vi "Shutdown.vi"(8 "error in (no error)":errorcluster, 11 "Nominal Streaming in":refnum<class "Stream.lvclass">) -> (0 "error out":errorcluster, 3 "Nominal Streaming out":refnum<class "Stream.lvclass">)   [LabVIEW 2020, in "Nominal Streaming.lvlib" / "Stream.lvclass"]
uses:
  Stream.lvclass
  Stream.lvclass/Stream.ctl
  bin/lib_nominal-streaming-lv_64.dll
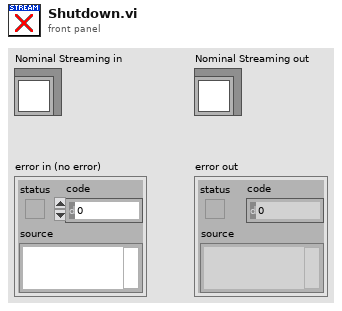
[diagram p1: front panel]
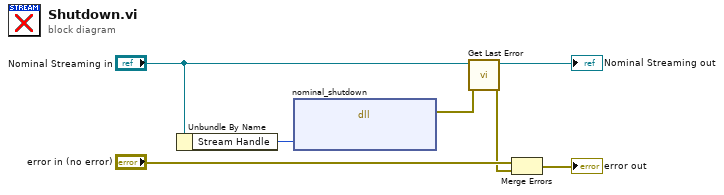
[diagram p0: block diagram]
diagram:
  n1 = Unbundle By Name("Nominal Streaming in") -> ("Stream Handle"=w7:u64)
  n2 = dll-call lib="C:/code/nominal-streaming-labview-ffi/lv_src/bin/lib_nominal-streaming-lv_*.*" fn="nominal_shutdown"("stream_handle"=w7) -> (error out=w6:errorcluster)  [unwired: 5 in, 1 out]
  n3 = call "Get Last Error.vi"("error in (no error)"=w6, "Nominal Streaming in"="Nominal Streaming in") -> ("error out"=w2:errorcluster, "Nominal Streaming out"=→"Nominal Streaming out":refnum<class "Stream.lvclass">)  [unwired: 8 in]
  n4 = Merge Errors("error in (no error)", w2) -> (→"error out":errorcluster)
